vi "Digital - Continuous Output_0207.vi"() -> ()   [LabVIEW 2021]
doc: "This example demonstrates how to continuously re-generate digital output data. That output is hardware timed, so each sample is output on the next tick of the sample clock.\n\nSome hardware (e.g. M Series DAQ) must use an external sample clock for digital tasks. To view a complete list of available sample clock sources, consult the Device Routes table in Measurement and Automation Explorer.\n\nFor instructions on how to connect your signals to the DAQ device, refer to your device documentation."
uses:
  <vilib>/Utility/error.llb/DialogType.ctl
  <vilib>/DAQmx/write.llb/DAQmx Write (Digital 1D U32 1Chan NSamp).vi
  <vilib>/DAQmx/create/channels.llb/DAQmx Create Channel (DO-Digital Output).vi
  <vilib>/DAQmx/configure/timing.llb/DAQmx Timing (Sample Clock).vi
  <vilib>/DAQmx/miscellaneous.llb/DAQmx Fill In Error Info.vi
  <resource>/objmgr/daqmx.rc
  <vilib>/DAQmx/configure/system.llb/DAQmx Set Power Up States (Digital).vi
panel:
  in  "Knob":dbl(knob) scale=0.0..10.0
  out "Time Pass per Loop":u32
  in  "stop (F)":bool
  in  "Line(s)":tag="Dev1/port0/line0:7"
  in  "Number of Samples":i32=1000
  in  "Sample Rate":dbl=1000.0
  in  "Sample Clock Source":tag="PFI0"
  out "Actual Sample Rate":dbl=1000.0 format="%0.2f"
  # "Channel Settings"
  # "Data to Write"
  # "Timing and Buffer Settings"
  # "Trigger Settings"
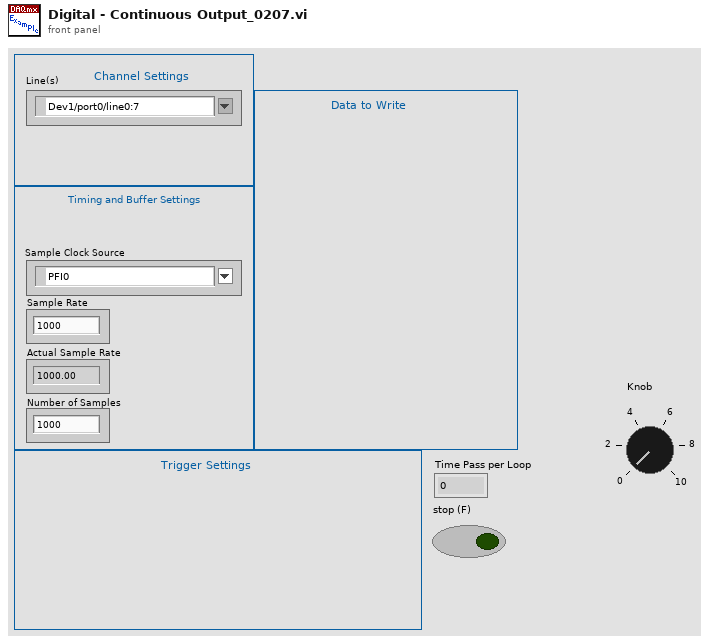
[diagram p1: front panel]
types:
  T1 = typedef "DialogType.ctl" = u16
  T2 = cluster{"physical channel":tag, "power up state":u16}[]
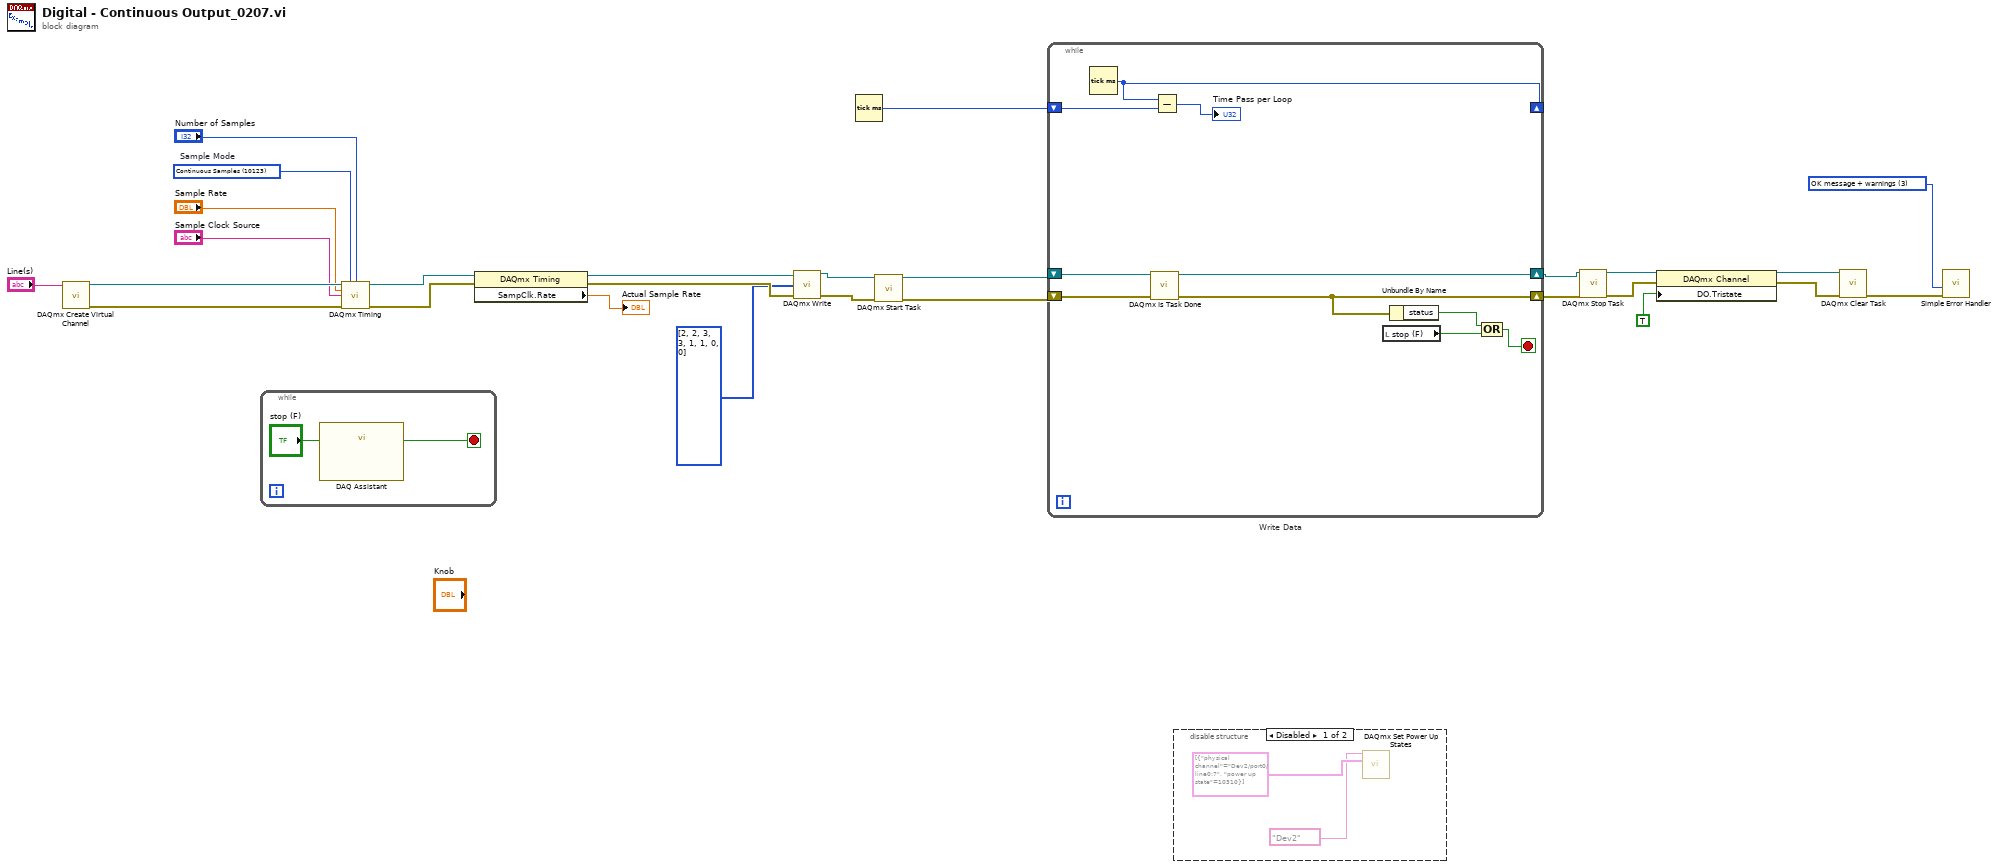
[diagram p0: block diagram]
diagram:
  w4 = 10123 items=["Finite Samples"=10178, "Continuous Samples"=10123, "Hardware Timed Single Point"=12522]  # Sample Mode
  w23 = T1 3 items=["no dialog", "OK message", "continue or stop message", "OK message + warnings", "continue/stop + warnings"] ("type of dialog (OK msg:1)")
  # "Write Data"
  n1 = call-poly <vilib>:"DAQmx Create Virtual Channel.vi"("lines"="Line(s)") -> ("task out"=w15:refnum<k21>, "error out"=w14:errorcluster)  [unwired: 13 in]
  n2 = while {
    stop <- w28 stop-if-true
    n3 = call "DAQ Assistant"("stop (F)"="stop (F)") -> ("stopped"=w28:bool)  [unwired: 16 in, 2 out]
  }
  n4 = call-poly <vilib>:"DAQmx Timing.vi"("task/channels in"=w15, "sample mode"=w4, "samples per channel"="Number of Samples", "rate"="Sample Rate", "source"="Sample Clock Source", "error in"=w14) -> ("task out"=w27:refnum<k21>, "error out"=w26:errorcluster)  [unwired: 8 in]
  n5 = property class="DAQmx Timing"(reference=w27, error in=w26) -> (reference out=w21:refnum<k21>, error out=w20:errorcluster, "SampClk.Rate"=→"Actual Sample Rate":dbl)
  n6 = call-poly <vilib>:"DAQmx Write.vi"("task/channels in"=w21, "data"=u32[] [2, 2, 3, 3, 1, 1, 0, 0], "error in"=w20) -> ("task out"=w19:refnum<k21>, "error out"=w18:errorcluster)  [unwired: 10 in, 1 out]
  n7 = Tick Count (ms)() -> (millisecond timer value=w22:u32)
  n8 = call <vilib>:"DAQmx Start Task.vi"("task/channels in"=w19, "error in"=w18) -> ("task out"=w17:refnum<k21>, "error out"=w16:errorcluster)  [unwired: 12 in]
  n9 = while {
    shift-right: [w34] -> w12
    shift-left: w17 -> [w36]
    shift-right: [w32] -> w11
    shift-left: w16 -> [w35]
    shift-right: [w38] -> _
    shift-left: w22 -> [w39]
    stop <- w30 stop-if-true
    n10 = Tick Count (ms)() -> (millisecond timer value=w38:u32)
    n11 = call <vilib>:"DAQmx Is Task Done.vi"("task/channels in"=w36, "error in"=w35) -> ("task out"=w34:refnum<k21>, "error out"=w32:errorcluster)  [unwired: 11 in, 1 out]
    n12 = Subtract(x=w38, y=w39) -> (x-y=→"Time Pass per Loop":u32)
    n13 = local read "stop (F)"() -> (w33:bool)
    n14 = Unbundle By Name(w32) -> ("status"=w31:bool)
    n15 = Compound Arithmetic op=OR(w31, w33) -> (w30:bool)
  }
  n16 = disable-structure shown="Disabled" {
    frame Disabled {
      n17 = call-poly <vilib>:"DAQmx Set Power Up States.vi"("device in"=tag "Dev2", "power up states"=T2 [{"physical channel"="Dev2/port0/line0:7", "power up state"=10310}]) -> ()  [unwired: 12 in, 2 out]
    }
    frame Enabled {
    }
  }
  n18 = call <vilib>:"DAQmx Stop Task.vi"("task/channels in"=w12, "error in"=w11) -> ("task out"=w10:refnum<k21>, "error out"=w9:errorcluster)  [unwired: 12 in]
  n19 = property class="DAQmx Channel"(reference=w10, error in=w9, "DO.Tristate"=TRUE) -> (reference out=w8:refnum<k21>, error out=w7:errorcluster)
  n20 = call <vilib>:"DAQmx Clear Task.vi"("task in"=w8, "error in"=w7) -> ("error out"=w1:errorcluster)  [unwired: 13 in]
  n21 = call <vilib>:"Simple Error Handler.vi"("type of dialog (OK msg:1)"=w23, "error in (no error)"=w1) -> ()  [unwired: 3 in, 5 out]
